vi "C867_Init.vi"(8 "error in":errorcluster caption="entrée d'erreur") -> (0 "error out":errorcluster caption="sortie d'erreur")   [LabVIEW 2026]
uses:
  C867-VIs/Low Level/Communication/Interface Settings.ctl
  Controls/TypeDef_FGV.ctl
panel:
  out "Position":dbl[](array[numeric]) format="%.6f"
  out "+/- movement\nrange":dbl[](array[numeric]) format="%.6f"
  out "Referenced?":bool[](array[boolean])
  out "Conn. Axis":string[](array[string])
  in  "Interface settings":T1={"Interface"=4, "Timeout"=5000, "RS232 settings"={"Portnumber"=1, "Baudrate"=5}, "TCP/IP settings"={"Host address/name"="localhost", "Port"=50000, "Board"=0, "TCP/IP Search?"=TRUE}, "USB settings"={"S/N"="", "USB Search?"=TRUE}, "DaisyChain settings"={"Register DC"=FALSE, "DaisyChain Search?"=TRUE, "Device ID"=1}, "DLL for Device"=0} {"DLL for Device" items=["None", "C-843", "C-844", "E-710", "C-843.PM", "C-865", "E-761", "Mercury", "E-755", "E-753", "C-866", "E-712", "E-725", "E-861", "C-867", "E-517", "E-816", "E-709", "PI_GCS2_DLL", "HydraPollux"]; "Interface" items=["RS232", "RS232 DaisyChain", "USB", "USB DaisyChain", "TCP/IP", "TCP/IP DaisyChain", "PCI"]; "RS232 settings"."Portnumber" min=1 step=1; "RS232 settings"."Baudrate" items=["9600", "14400", "19200", "38400", "57600", "115200", "230400", "460800"]}
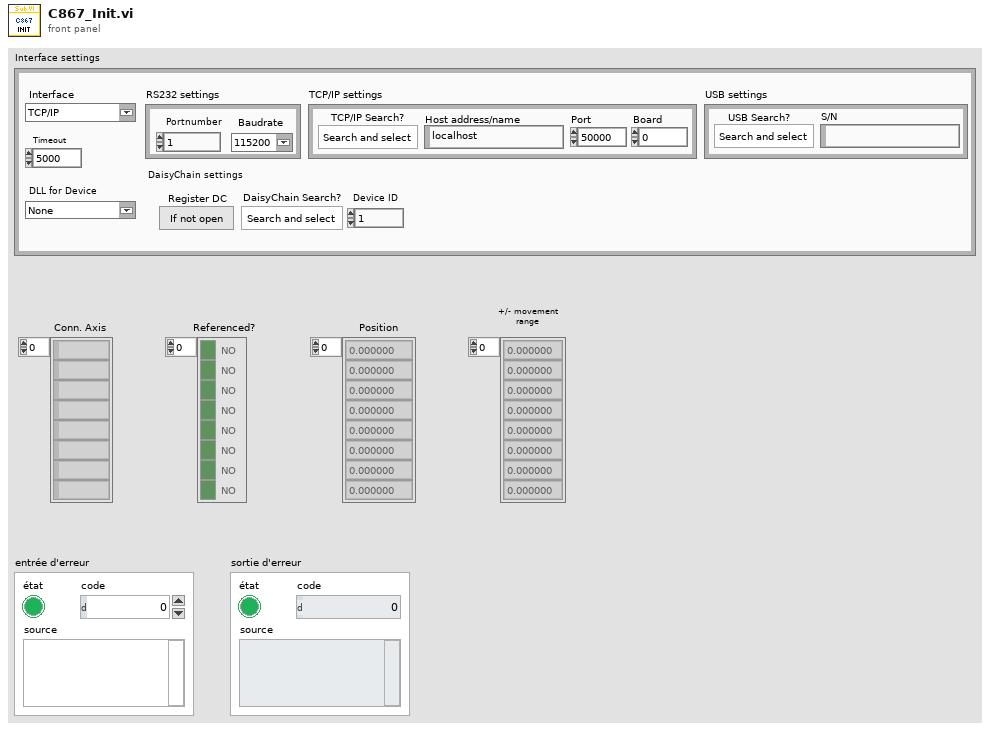
[diagram p1: front panel]
types:
  T1 = typedef "Interface Settings.ctl" = cluster{"Interface":u16, "Timeout":u32, "RS232 settings":cluster{"Portnumber":u8, "Baudrate":u16}, "TCP/IP settings":cluster{"Host address/name":string, "Port":i32, "Board":i32, "TCP/IP Search?":bool}, "USB settings":cluster{"S/N":string, "USB Search?":bool}, "DaisyChain settings":cluster{"Register DC":bool, "DaisyChain Search?":bool, "Device ID":i32}, "DLL for Device":u16}
  T2 = typedef "TypeDef_FGV.ctl" = enum16{"Initialize", "Write", "Read"}
  T3 = enum16{"Do not reference", "Reference switch", "Negative limit switch", "Positive limit switch"}[]
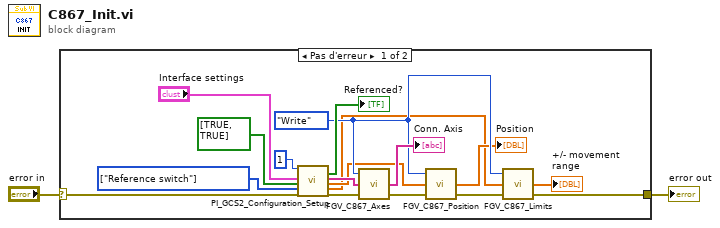
[diagram p0: block diagram]
diagram:
  n1 = case shown="Pas d'erreur" "error in" {
    selector: "error in" -> [w19 w20]
    tunnel: [w10 w20] -> w1
    frame No Error {
      w7 = TypeDef_FGV."Write" ("Action")
      w16 = T3 [enum."Reference switch"] items=["Do not reference", "Reference switch", "Negative limit switch", "Positive limit switch"] ("Reference mode")
      n2 = call "PI_GCS2_Configuration_Setup.vi"("System no."=1, "Interface settings"="Interface settings", "Closed Loop"=bool[] [TRUE, TRUE], "Reference mode"=w16, "error in"=w19) -> ("Referenced?"=→"Referenced?":bool[], "Conn. Axis"=w9:string[], "Position"=w6:dbl[], "+/- movement\nrange"=w4:dbl[], "error out"=w13:errorcluster)  [unwired: 9 in, 1 out]
      n3 = call "FGV_C867_Axes.vi"("error in"=w13, "Conn. Axis"=w9, "Action"=w7) -> ("error out"=w12:errorcluster, "Conn. Axis"=→"Conn. Axis":string[])  [unwired: 1 in]
      n4 = call "FGV_C867_Position.vi"("error in"=w12, "Position"=w6, "Action"=w7) -> ("error out"=w11:errorcluster, "Position"=→"Position":dbl[])  [unwired: 1 in]
      n5 = call "FGV_C867_Limits.vi"("error in"=w11, "Limits"=w4, "Action"=w7) -> ("error out"=w10:errorcluster, "Limits"=→"+/- movement\nrange":dbl[])  [unwired: 1 in]
    }
    frame Error {
    }
  }
  "error out" <- w1
